vi "main.vi"(11 "client class":refnum<class "client.lvclass">) -> ()   [LabVIEW 2020, in "client.lvclass"]
uses:
  client.lvclass
  shared/message--cluster.ctl
  shared/request--enum.ctl
  client.lvclass/client.ctl
  shared/_JKI_lib_State_Machine.llb/Select State(s)_err__jki_lib_state_machine.vi
panel:
  out "value":T1
  out "error out":errorcluster[](array[cluster])
  in  "Exit":bool
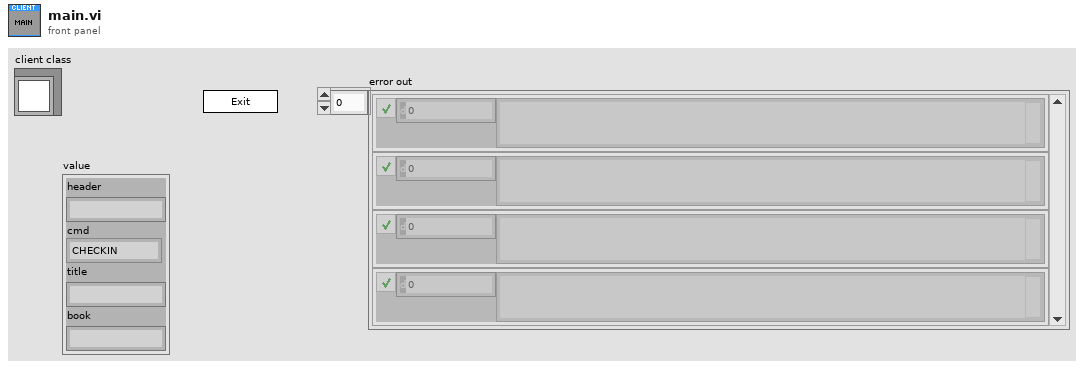
[diagram p1: front panel]
types:
  T1 = typedef "message--cluster.ctl" = cluster{"header":string, "cmd":T2, "title":string, "book":string}
  T2 = typedef "request--enum.ctl" = enum16{"CHECKIN", "CHECKOUT"}
  T3 = enum32{"Invalid", "Standard", "Closed", "Hidden", "Minimized", "Maximized"}
  T4 = enum32{"invalid app kind", "Development System", "Run Time System", "Student Edition", "Embedded LabVIEW", "Evaluation", "Custom"}
  T5 = cluster{"Core":cluster{"Current VI Reference":refnum<vi>, "Close Panel on Exit?":bool}, "client class":refnum<class "client.lvclass">, "TO":i32, "tcp ref":refnum<k5>, "UUID":string, "Book Text":string}
  T6 = cluster{"Current VI Reference":refnum<vi>, "Close Panel on Exit?":bool}
  T7 = cluster{"exit event":refnum<user-event>, "checkout event":refnum<user-event>, "checkin event":refnum<user-event>, "damage event":refnum<user-event>}
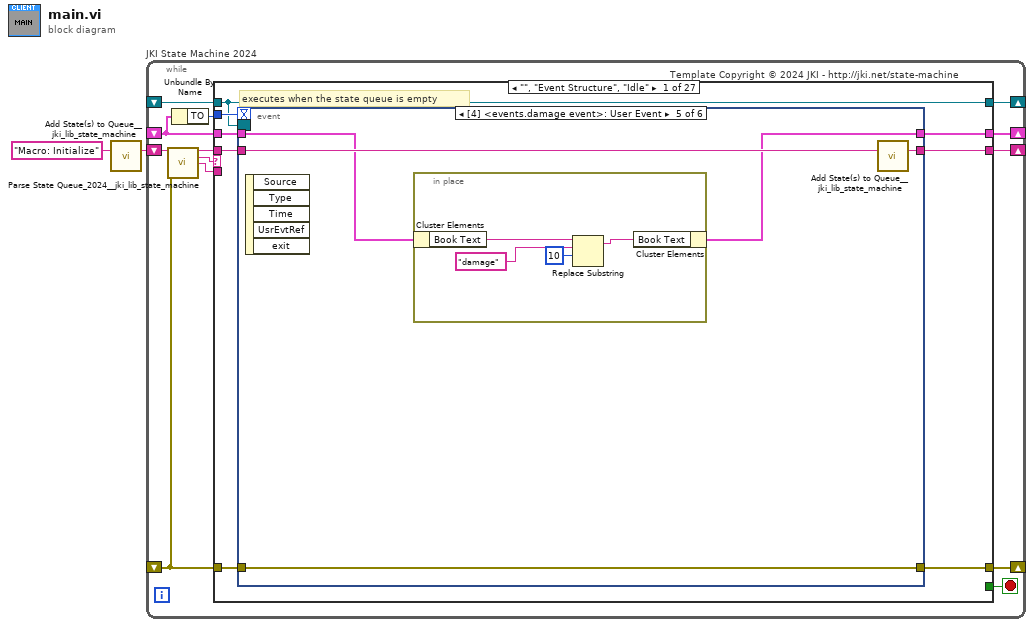
[diagram p0: block diagram]
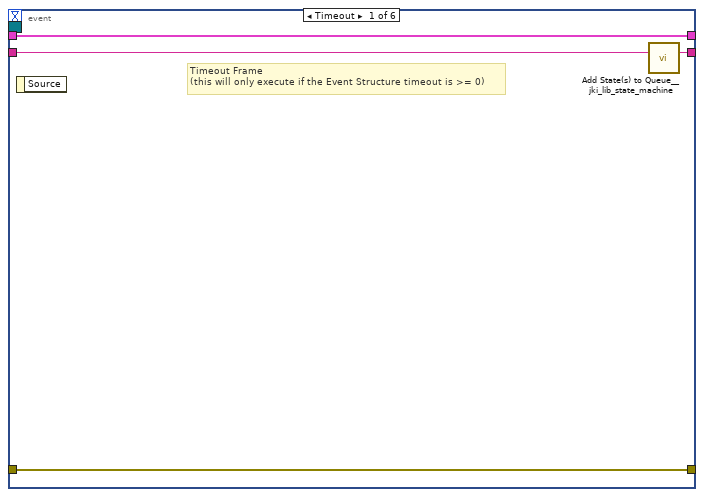
[diagram p2: hidden frame]
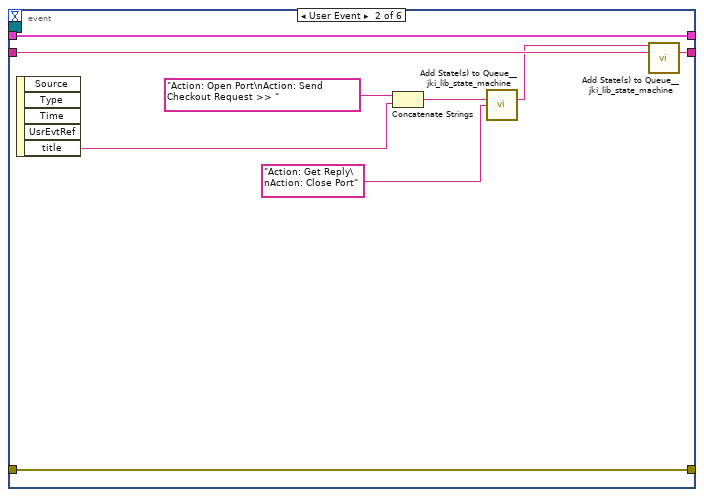
[diagram p3: hidden frame]
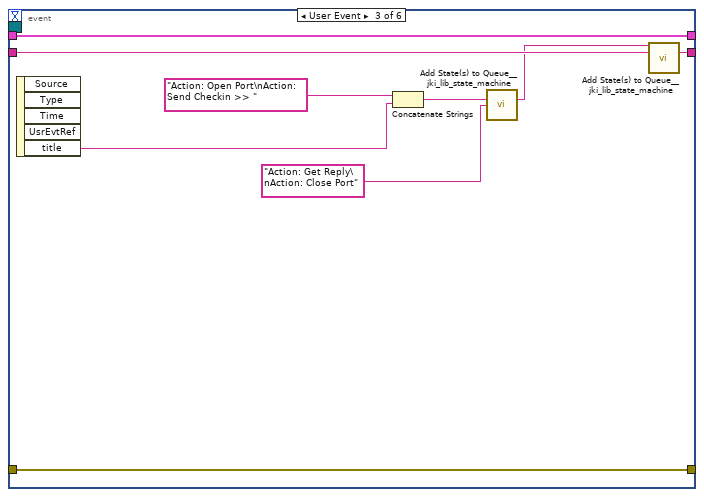
[diagram p4: hidden frame]
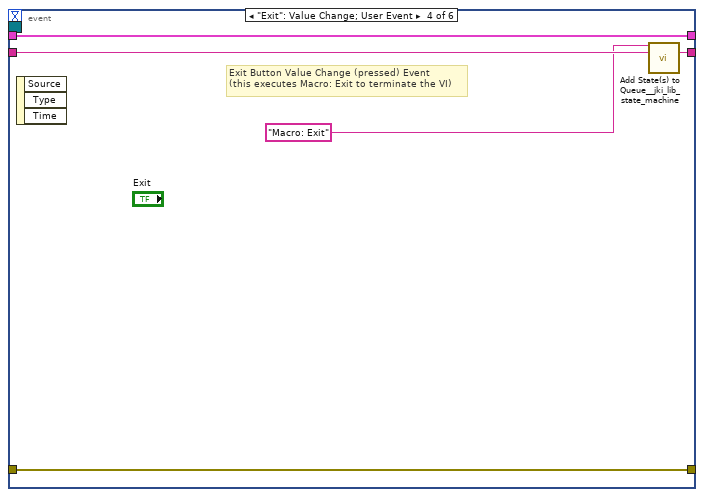
[diagram p5: hidden frame]
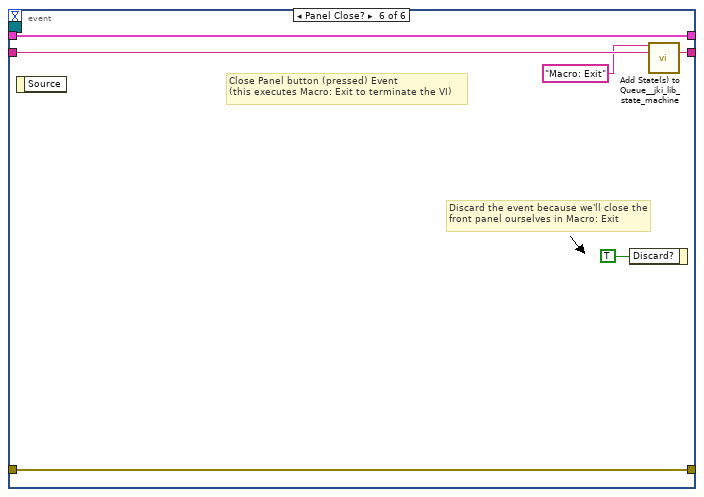
[diagram p6: hidden frame]
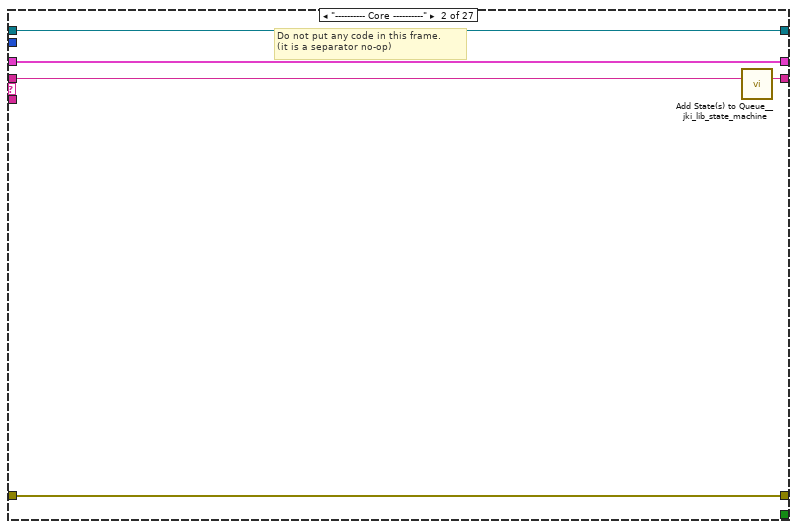
[diagram p7: hidden frame]
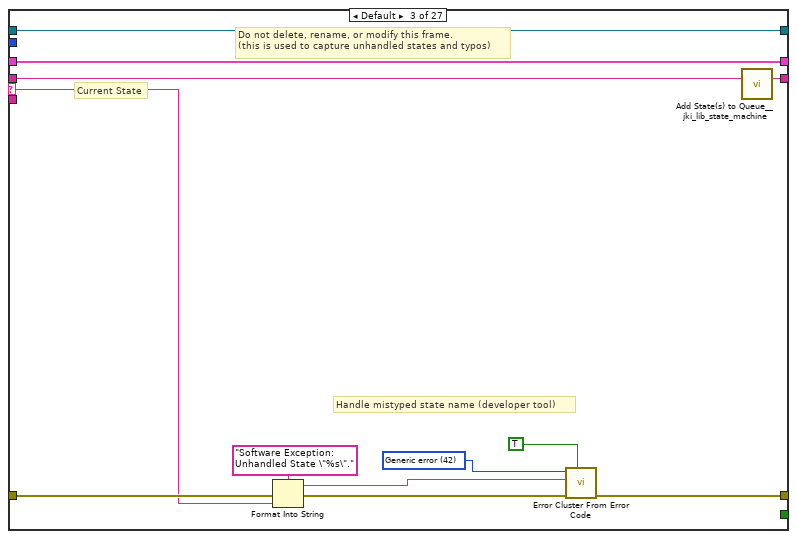
[diagram p8: hidden frame]
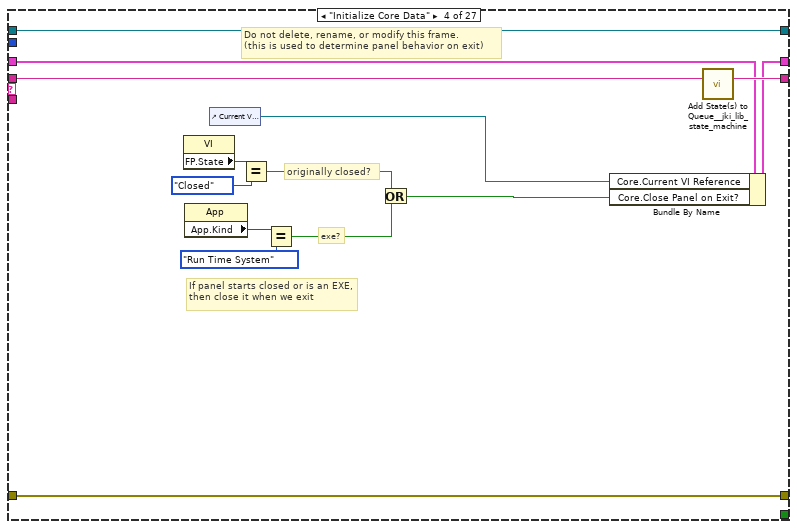
[diagram p9: hidden frame]
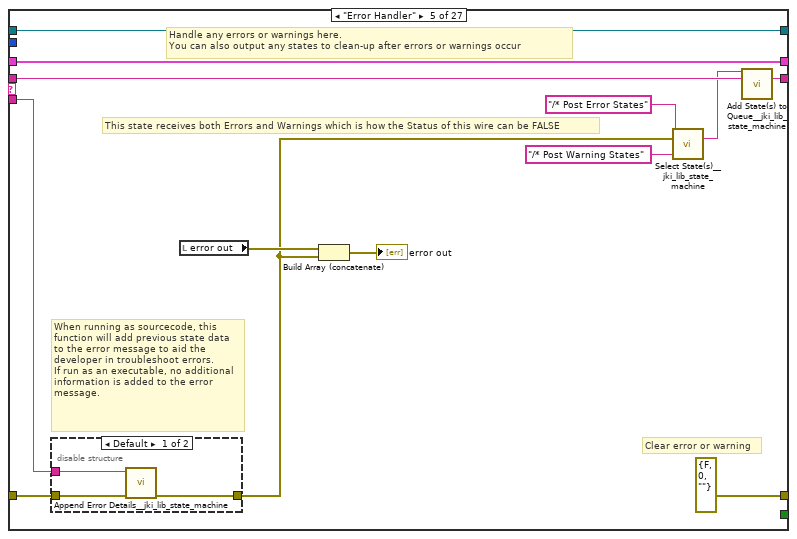
[diagram p10: hidden frame]
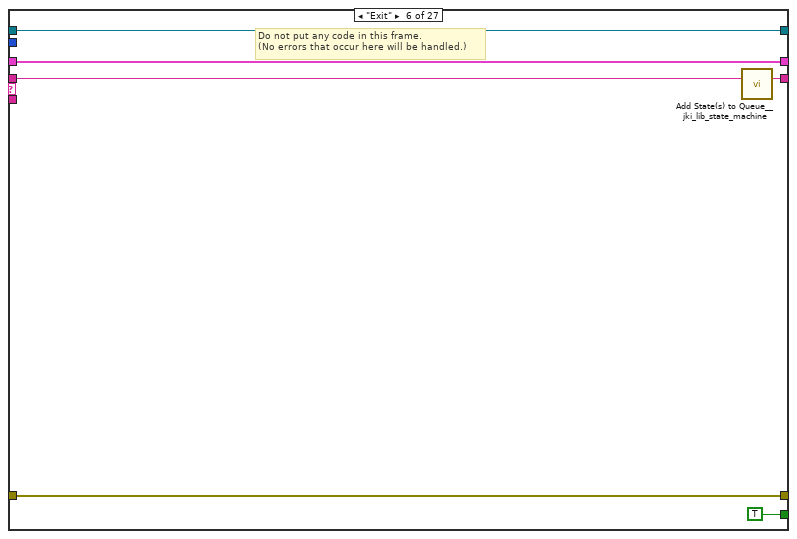
[diagram p12: hidden frame]
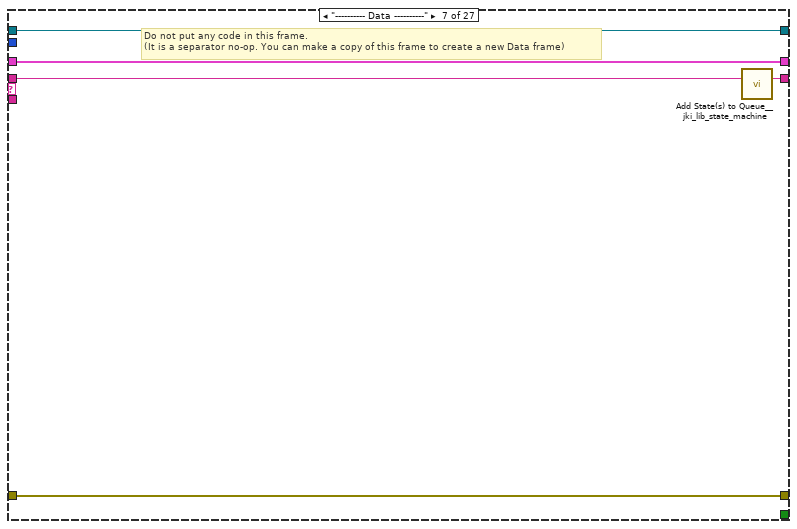
[diagram p13: hidden frame]
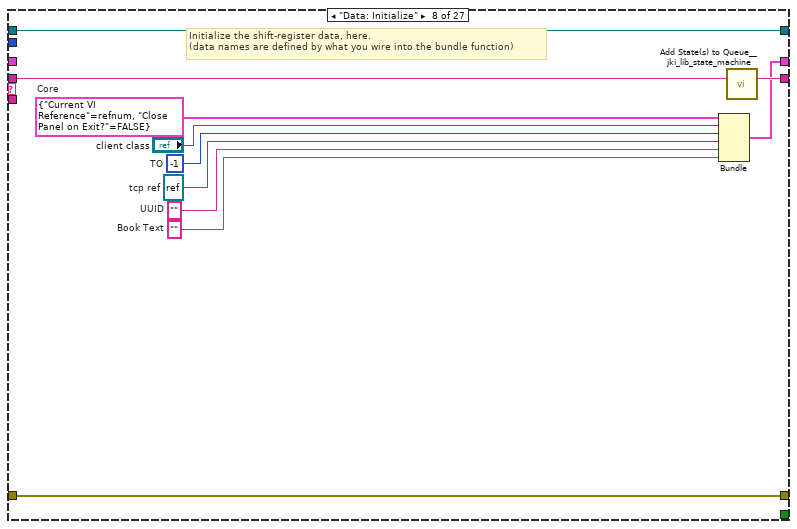
[diagram p14: hidden frame]
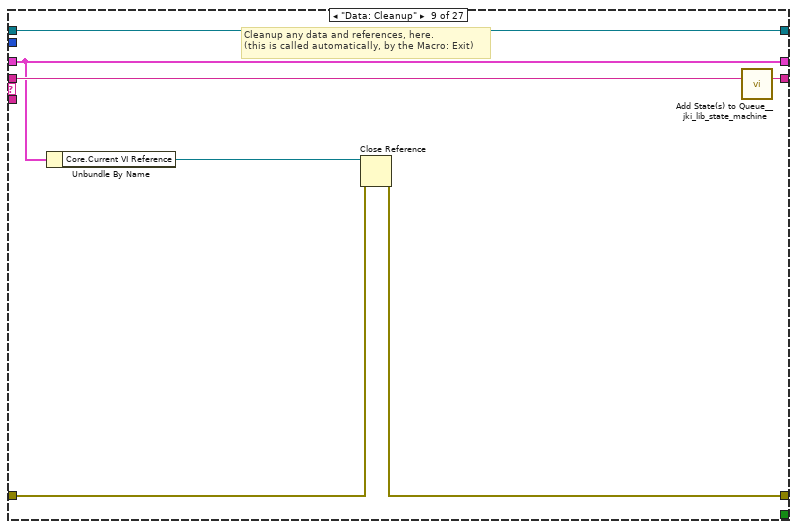
[diagram p15: hidden frame]
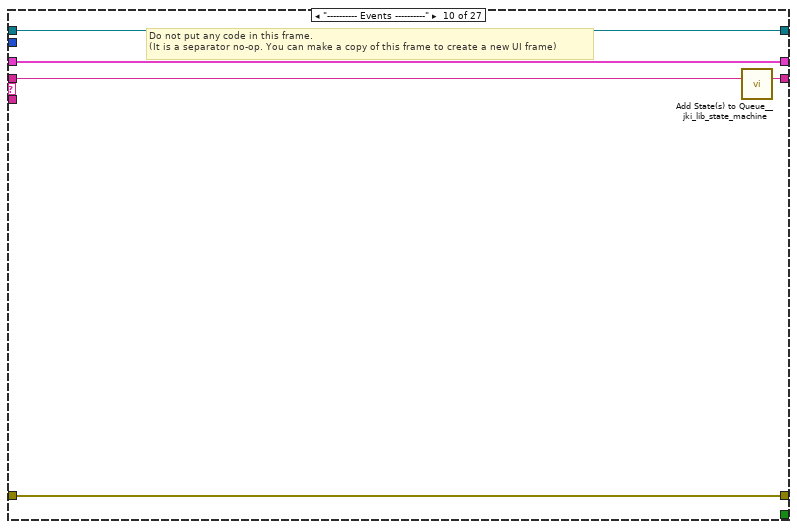
[diagram p16: hidden frame]
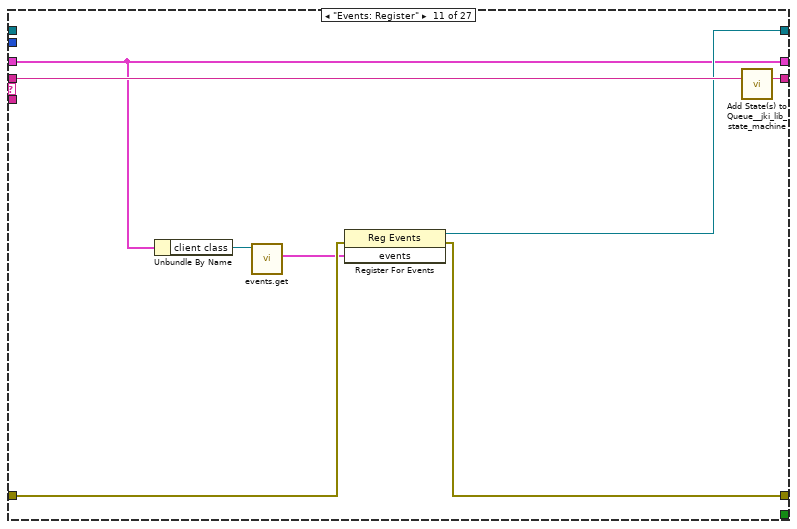
[diagram p17: hidden frame]
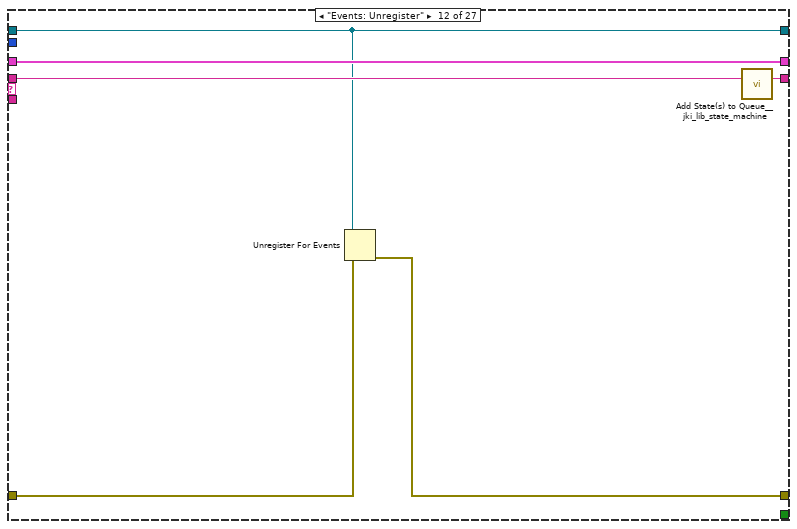
[diagram p18: hidden frame]
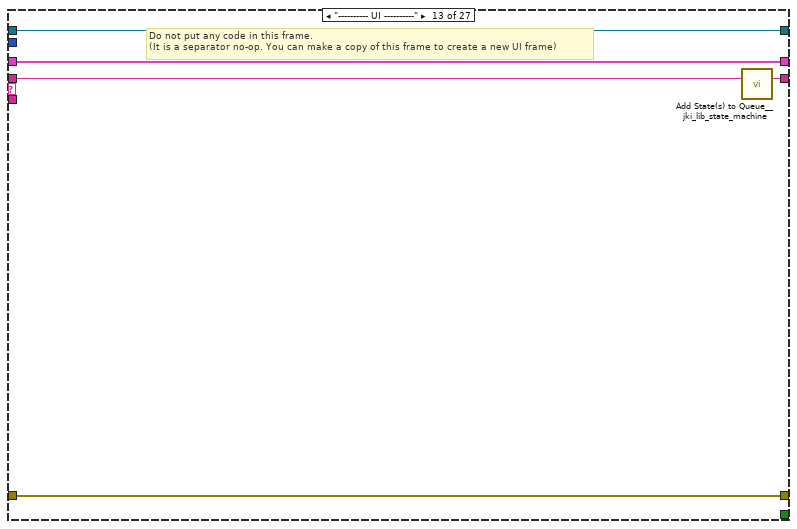
[diagram p19: hidden frame]
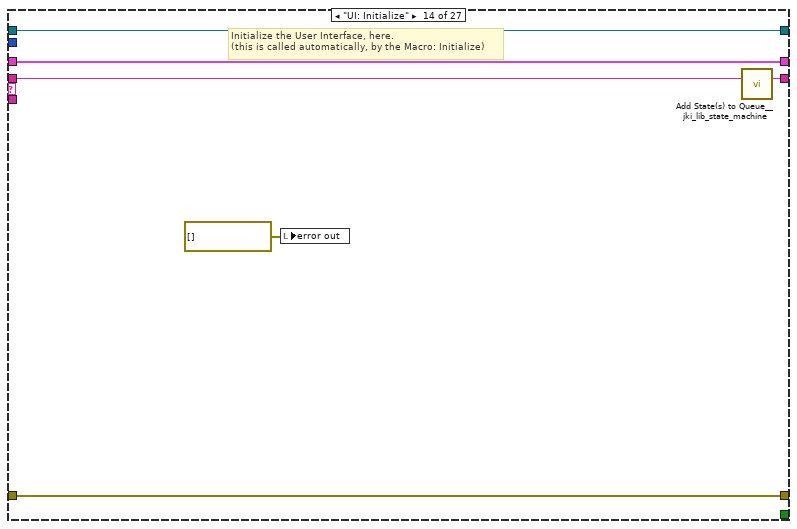
[diagram p20: hidden frame]
diagram:
  n1 = call "Add State(s) to Queue__jki_lib_state_machine.vi"("State(s) in (\"\")"="Macro: Initialize") -> ("States Out"=w2:string)  [unwired: 14 in]
  n2 = while "JKI State Machine 2024" {
    shift-right: [w8] -> _
    shift-left: _ -> [w4]
    shift-right: [w11] -> _
    shift-left: _ -> [w7]
    shift-right: [w10] -> _
    shift-left: w2 -> [w12]
    shift-right: [w6] -> _
    shift-left: _ -> [w5]
    stop <- w9 stop-if-true
    # "Template Copyright © 2024 JKI - http://jki.net/state-machine"
    n3 = call "Parse State Queue_2024__jki_lib_state_machine.vi"("State Queue"=w12, "Error In (no error)"=w7) -> ("Remaining States"=w14:string, "Current State"=w15:string, "Arguments"=w13:string)  [unwired: 11 in]
    n4 = Unbundle By Name(w4) -> ("TO"=w3:i32)
    n5 = case shown="\"\", \"Event Structure\", \"Idle\"" w15 {
      selector: w15 -> [_ _ w72 _ _ _ _ _ _ _ _ _ _ _ _ _ _ _ _ _ _ _ _ _ _ _ _]
      tunnel: w14 -> [w23 w70 w76 w96 w109 w119 w124 w135 w142 w147 w155 w161 w166 w172 w177 w184 w196 w266 w272 w282 w287 w308 w316 w326 w333 w350 w368]
      tunnel: w13 -> [_ _ _ _ w104 _ _ _ _ _ _ _ _ _ _ w179 w190 _ _ _ _ _ _ _ _ w342 w361]
      tunnel: w4 -> [w21 w67 w74 w89 w106 w117 w121 _ w137 w144 w150 w159 w163 w170 w175 w182 w192 w263 w269 w280 w284 w291 w311 w319 w330 w347 w351]
      tunnel: [w20 w68 w78 w93 errorcluster {"status"=FALSE, "code"=0, "source"=""} ("error out") w116 w122 w132 w138 w145 w151 w156 w164 w169 w174 w180 w193 w264 w270 w277 w285 w292 w312 w320 w327 w338 w357] -> w11
      tunnel: w7 -> [w17 w68 w77 w93 w105 w116 w122 w132 w139 w145 w152 w157 w164 w169 w174 w181 w194 w264 w270 w277 w285 w295 w313 w321 w328 w340 w359]
      tunnel: [w22 w69 w75 w95 w108 w118 w123 w134 w141 w146 w154 w160 w165 w171 w176 w183 w195 w265 w271 w281 w286 w307 w315 w325 w332 w349 w367] -> w10
      tunnel: [_ _ _ _ _ TRUE _ _ _ _ _ _ _ _ _ _ _ _ _ _ _ _ _ _ _ _ _] -> w9
      tunnel: [w19 w67 w74 w94 w106 w117 w121 w133 w137 w144 w150 w159 w163 w170 w175 w182 w192 w263 w269 w280 w284 w290 w310 w318 w330 w347 w351] -> w8
      tunnel: w3 -> [w18 _ _ _ _ _ _ _ _ _ _ _ _ _ _ _ _ _ _ _ _ _ _ _ _ _ _]
      tunnel: [w16 w66 w71 w83 w100 w114 w120 w130 w136 w143 w153 w158 w162 w168 w173 w178 w189 w262 w267 w273 w283 w306 w314 w324 w331 w348 w366] -> w6
      tunnel: w5 -> [w16 w66 w71 w83 w100 w114 w120 w130 w136 w143 _ w158 w162 w168 w173 w178 w189 w262 w267 w273 w283 w306 w314 w324 w331 w348 w366]
      frame "", "Event Structure", "Idle" {
        # "executes when the state queue is empty"
        n6 = event shown="[4] <events.damage event>: User Event" {
          selector: w16 -> [_ _ _ _ _ _]
          dyn-events: _ -> [_ _ _ _ _ _]
          timeout: w18 -> [_ _ _ _ _ _]
          tunnel: w23 -> [w27 w36 w45 w50 w55 w65]
          tunnel: [w26 w35 w44 w49 w54 w64] -> w22
          tunnel: w21 -> [w24 w33 w42 w47 w52 w62]
          tunnel: [w25 w34 w43 w48 w53 w63] -> w20
          tunnel: w17 -> [w25 w34 w43 w48 w53 w63]
          tunnel: [w24 w33 w42 w47 w51 w62] -> w19
          event Timeout {
            # "Timeout Frame\n(this will only execute if the Event Structure timeout is >= 0)"
            n7 = event-data() -> ()  [unwired: 1 in, 1 out]
            n8 = call "Add State(s) to Queue__jki_lib_state_machine.vi"("State(s) in (\"\")"=w27) -> ("States Out"=w26:string)  [unwired: 14 in]
          }
          event User Event {
            n9 = event-data() -> ("title"=w31:string)  [unwired: 1 in, 4 out]
            n10 = Concatenate Strings("Action: Open Port\nAction: Send Checkout Request >> ", w31) -> (w30:string)
            n11 = call "Add State(s) to Queue__jki_lib_state_machine.vi"("State(s) in (\"\")"=w30, "State(s) at Back (\"\")"="Action: Get Reply\nAction: Close Port") -> ("States Out"=w28:string)  [unwired: 13 in]
            n12 = call "Add State(s) to Queue__jki_lib_state_machine.vi"("State(s) in Front (\"\")"=w28, "State(s) in (\"\")"=w36) -> ("States Out"=w35:string)  [unwired: 13 in]
          }
          event User Event {
            n13 = event-data() -> ("title"=w40:string)  [unwired: 1 in, 4 out]
            n14 = Concatenate Strings("Action: Open Port\nAction: Send Checkin >> ", w40) -> (w39:string)
            n15 = call "Add State(s) to Queue__jki_lib_state_machine.vi"("State(s) in (\"\")"=w39, "State(s) at Back (\"\")"="Action: Get Reply\nAction: Close Port") -> ("States Out"=w37:string)  [unwired: 13 in]
            n16 = call "Add State(s) to Queue__jki_lib_state_machine.vi"("State(s) in Front (\"\")"=w37, "State(s) in (\"\")"=w45) -> ("States Out"=w44:string)  [unwired: 13 in]
          }
          event "Exit": Value Change; User Event {
            # "Exit Button Value Change (pressed) Event\n(this executes Macro: Exit to terminate the VI)"
            n17 = event-data() -> ()  [unwired: 1 in, 3 out]
            n18 = call "Add State(s) to Queue__jki_lib_state_machine.vi"("State(s) in Front (\"\")"="Macro: Exit", "State(s) in (\"\")"=w50) -> ("States Out"=w49:string)  [unwired: 13 in]
          }
          event User Event {
            n19 = event-data() -> ()  [unwired: 1 in, 5 out]
            n20 = in-place {
              n21 = in-place-cluster #1(w52) -> ("Book Text"=w59:string)
              n22 = Replace Substring(3:10 ("offset (0)"), 4:"damage" ("substring (\"\")"), 5:w59) -> (1:w57:string)  [unwired: 1 in, 1 out]
              n23 = in-place-cluster #1("Book Text"=w57) -> (w51:T5)
            }
            n24 = call "Add State(s) to Queue__jki_lib_state_machine.vi"("State(s) in (\"\")"=w55) -> ("States Out"=w54:string)  [unwired: 14 in]
          }
          event Panel Close? {
            # "Discard the event because we'll close the front panel ourselves in Macro: Exit"
            # "Close Panel button (pressed) Event\n(this executes Macro: Exit to terminate the VI)"
            n25 = event-data() -> ()  [unwired: 1 in, 1 out]
            n26 = event-data("Discard?"=TRUE) -> ()  [unwired: 1 in, 1 out]
            n27 = call "Add State(s) to Queue__jki_lib_state_machine.vi"("State(s) in Front (\"\")"="Macro: Exit", "State(s) in (\"\")"=w65) -> ("States Out"=w64:string)  [unwired: 13 in]
          }
        }
      }
      frame "---------- Core ----------" {
        # "Do not put any code in this frame.\n(it is a separator no-op)"
        n28 = call "Add State(s) to Queue__jki_lib_state_machine.vi"("State(s) in (\"\")"=w70) -> ("States Out"=w69:string)  [unwired: 14 in]
      }
      frame Default {
        w81 = 42 items=["No error", "Argument error", "Memory is full", "Out of zone", "End of file", "File already open", "Generic file I/O error", "File not found", "File permission error", "Disk is full", "Duplicate path", "Too many files open", "System feature not enabled", "Resource file not found", "Cannot add resource", "Resource not found", "Image not found", "Image memory error", "Pen does not exist", "Config type invalid", "Config token not found", "Config parse error", "Config memory error", "Bad external code format", "Bad external code offset", "External code not present", "Null window", "Destroy window error", "Null menu", "Print aborted", "Bad print record", "Print driver error", "Windows error during printing", "Memory error during printing", "Print dialog error", "Generic print error", "Invalid device refnum", "Device not found", "Device parameter error", "Device unit error", "Cannot open device", "Device call aborted", "Generic error", "Cancelled by user", "Object ID too low", "Object ID too high", "Object not in heap", "Unknown heap", "Unknown object (invalid DefProc)", "Unknown object (DefProc not in table)", "Message out of range", "Invalid (null) method", "Unknown message", "Manager call not supported", "Bad address", "Network operation in progress", "Network operation timed out", "Connection is busy", "Network attribute not supported", "Network error", "Address in use", "System out of memory", "Connection aborted", "Connection refused", "Not connected", "Already connected", "Connection closed", "Initialization error (interapplication manager)", "Bad occurrence", "Wait on unbound occurrence handler", "Occurrence queue overflow", "Datalog type conflict", "Unused", "Unrecognized type (interapplication manager)", "Memory corrupt", "Failed to make temporary DLL", "Old CIN version", "Drag socket not found", "Failed to load drop-object", "Failed to register OLE object", "Failed to release OLE object", "Format specifier type mismatch", "Unknown format specifier", "Too few format specifiers", "Too many format specifiers", "Scan failed", "Newer CIN version", "Error converting to variant", "Runtime menu error", "Password tampered", "Variant attribute not found", "Incompatible variant data type", "Event data is not available", "Event Store is not present", "Occurrence is not found", "Event Queue is not created", "Event info is not available", "Refnum passed is NULL", "Error retrieving Class GUID", "Error retrieving CoClass GUID", "Error retrieving TypeLib GUID.", "Bad built application magic bytes.", "Specific driver is different from the specific driver associated with the Logical Name.", "There is no session opened to the class driver.", "Max Error", "MAX - Error with config objects", "MAX - Error loading configuration", "MAX - Group not supported"]
        # "Current State"
        # "Do not delete, rename, or modify this frame.\n(this is used to capture unhandled states and typos)"
        # "Handle mistyped state name (developer tool)"
        n29 = Format Into String(format string="Software Exception: Unhandled State \"%s\"." ("message"), error in=w77, w72) -> (resulting string=w80:string, error out=w79:errorcluster)  [unwired: 1 in]
        n30 = call <vilib>:"Error Cluster From Error Code.vi"("show call chain? (False)"=TRUE, "error in (no error)"=w79, "error message (\"\")"=w80, "error code (0)"=w81) -> ("error out"=w78:errorcluster)  [unwired: 5 in]
        n31 = call "Add State(s) to Queue__jki_lib_state_machine.vi"("State(s) in (\"\")"=w76) -> ("States Out"=w75:string)  [unwired: 14 in]
      }
      frame "Initialize Core Data" {
        # "Do not delete, rename, or modify this frame.\n(this is used to determine panel behavior on exit)"
        # "originally closed?"
        # "exe?"
        # "If panel starts closed or is an EXE, then close it when we exit"
        n32 = property class="VI"() -> ("FP.State"=w86:T3)  [unwired: 2 in, 2 out]
        n33 = property class="App"() -> ("App.Kind"=w92:T4)  [unwired: 2 in, 2 out]
        n34 = control-ref of="Current VI Reference"() -> (w87:refnum<vi>)
        n35 = Equal?(x=w86, y=T3."Closed" ("Front Panel Window:State")) -> (x = y?=w84:bool)
        n36 = Equal?(x=w92, y=T4."Run Time System" ("Application:Kind")) -> (x = y?=w90:bool)
        n37 = Or(x=w84, y=w90) -> (x .or. y?=w88:bool)
        n38 = Bundle By Name(cluster=w89, "Core.Current VI Reference"=w87, "Core.Close Panel on Exit?"=w88) -> (w94:T5)
        n39 = call "Add State(s) to Queue__jki_lib_state_machine.vi"("State(s) in (\"\")"=w96) -> ("States Out"=w95:string)  [unwired: 14 in]
      }
      frame "Error Handler" {
        # "When running as sourcecode, this function will add previous state data to the error message to aid the developer in troubleshoot errors.\nIf run as an executable, no additional information is added to the error message."
        # "This state receives both Errors and Warnings which is how the Status of this wire can be FALSE"
        # "Handle any errors or warnings here.\nYou can also output any states to clean-up after errors or warnings occur"
        # "Clear error or warning"
        n40 = disable-structure shown="Default" {
          disable-tunnel: w105 -> [w112 w113]
          disable-tunnel: w104 -> [w111 _]
          disable-tunnel: [w110 w113] -> w98
          frame condition #0 (active) {
            n41 = call "Append Error Details__jki_lib_state_machine.vi"("error in (no error)"=w112, "Previous State and Argument(s)"=w111) -> ("error out"=w110:errorcluster)  [unwired: 9 in]
          }
          frame condition #1 {
          }
        }
        n42 = local read "error out"() -> (w99:errorcluster[])
        n43 = Build Array (concatenate)(w99, w98) -> (→"error out":errorcluster[])
        n44 = call-poly "Select State(s)__jki_lib_state_machine.vi"("State(s) if True (\"\")"="/* Post Error States", "Select"=w98, "State(s) if False (\"\")"="/* Post Warning States") -> ("States Out"=w102:string)  [unwired: 12 in]
        n45 = call "Add State(s) to Queue__jki_lib_state_machine.vi"("State(s) in Front (\"\")"=w102, "State(s) in (\"\")"=w109) -> ("States Out"=w108:string)  [unwired: 13 in]
      }
      frame "Exit" {
        # "Do not put any code in this frame.\n(No errors that occur here will be handled.)"
        n46 = call "Add State(s) to Queue__jki_lib_state_machine.vi"("State(s) in (\"\")"=w119) -> ("States Out"=w118:string)  [unwired: 14 in]
      }
      frame "---------- Data ----------" {
        # "Do not put any code in this frame.\n(It is a separator no-op. You can make a copy of this frame to create a new Data frame)"
        n47 = call "Add State(s) to Queue__jki_lib_state_machine.vi"("State(s) in (\"\")"=w124) -> ("States Out"=w123:string)  [unwired: 14 in]
      }
      frame "Data: Initialize" {
        w125 = ""  # Book Text
        w126 = ""  # UUID
        w127 = refnum<k5> refnum  # tcp ref
        w128 = -1  # TO
        w131 = T6 {"Current VI Reference"=refnum, "Close Panel on Exit?"=FALSE}  # Core
        # "Initialize the shift-register data, here.\n(data names are defined by what you wire into the bundle function)"
        n48 = Bundle("Core"=w131, "client class"="client class", "TO"=w128, "tcp ref"=w127, "UUID"=w126, "Book Text"=w125) -> (w133:T5)  [unwired: 1 in]
        n49 = call "Add State(s) to Queue__jki_lib_state_machine.vi"("State(s) in (\"\")"=w135) -> ("States Out"=w134:string)  [unwired: 14 in]
      }
      frame "Data: Cleanup" {
        # "Cleanup any data and references, here.\n(this is called automatically, by the Macro: Exit)"
        n50 = Unbundle By Name(w137) -> ("Core.Current VI Reference"=w140:refnum<vi>)
        n51 = Close Reference(reference=w140, error in (no error)=w139) -> (error out=w138:errorcluster)
        n52 = call "Add State(s) to Queue__jki_lib_state_machine.vi"("State(s) in (\"\")"=w142) -> ("States Out"=w141:string)  [unwired: 14 in]
      }
      frame "---------- Events ----------" {
        # "Do not put any code in this frame.\n(It is a separator no-op. You can make a copy of this frame to create a new UI frame)"
        n53 = call "Add State(s) to Queue__jki_lib_state_machine.vi"("State(s) in (\"\")"=w147) -> ("States Out"=w146:string)  [unwired: 14 in]
      }
      frame "Events: Register" {
        n54 = Unbundle By Name(w150) -> ("client class"=w149:refnum<class "client.lvclass">)
        n55 = call "events.get.vi"("client in"=w149) -> ("events"=w148:T7)  [unwired: 9 in, 1 out]
        n56 = register-events(error in=w152, w148) -> (reference out=w153:refnum<event-registration>, error out=w151:errorcluster)  [unwired: 1 in]
        n57 = call "Add State(s) to Queue__jki_lib_state_machine.vi"("State(s) in (\"\")"=w155) -> ("States Out"=w154:string)  [unwired: 14 in]
      }
      frame "Events: Unregister" {
        n58 = Unregister For Events(event registration refnum=w158, error in=w157) -> (error out=w156:errorcluster)
        n59 = call "Add State(s) to Queue__jki_lib_state_machine.vi"("State(s) in (\"\")"=w161) -> ("States Out"=w160:string)  [unwired: 14 in]
      }
      frame "---------- UI ----------" {
        # "Do not put any code in this frame.\n(It is a separator no-op. You can make a copy of this frame to create a new UI frame)"
        n60 = call "Add State(s) to Queue__jki_lib_state_machine.vi"("State(s) in (\"\")"=w166) -> ("States Out"=w165:string)  [unwired: 14 in]
      }
      frame "UI: Initialize" {
        # "Initialize the User Interface, here.\n(this is called automatically, by the Macro: Initialize)"
        n61 = local write "error out"(errorcluster[] [] ("error out")) -> ()
        n62 = call "Add State(s) to Queue__jki_lib_state_machine.vi"("State(s) in (\"\")"=w172) -> ("States Out"=w171:string)  [unwired: 14 in]
      }
      frame "UI: Uninitialize" {
        # "Cleanup the User Interface, here.\n(this is called automatically, by the Macro: Exit)"
        n63 = call "Add State(s) to Queue__jki_lib_state_machine.vi"("State(s) in (\"\")"=w177) -> ("States Out"=w176:string)  [unwired: 14 in]
      }
      frame "UI: Cursor Set" {
        # "Argument"
        # "Set and Unset Cursor Busy.\n(Usage: \"UI: Cursor Set >> Busy|Idle\")"
        n64 = case shown="\"Idle\", Default" w179 {
          tunnel: w181 -> [w186 w188]
          tunnel: [w185 w187] -> w180
          frame "Idle", Default {
            n65 = call <vilib>:"Unset Busy.vi"("error in (no error)"=w186) -> ("error out"=w185:errorcluster)  [unwired: 10 in]
          }
          frame "Busy" {
            n66 = call <vilib>:"Set Busy.vi"("error in (no error)"=w188) -> ("error out"=w187:errorcluster)  [unwired: 9 in, 1 out]
          }
        }
        n67 = call "Add State(s) to Queue__jki_lib_state_machine.vi"("State(s) in (\"\")"=w184) -> ("States Out"=w183:string)  [unwired: 14 in]
      }
      frame "UI: Front Panel State" {
        # "Argument"
        # "Set Front Panel Open or Closed\n(Usage: \"UI: Front Panel State >> Open|Close\")"
        n68 = Unbundle By Name(w192) -> ("Core.Current VI Reference"=w191:refnum<vi>)
        n69 = case shown="\"Minimize\", \"Minimized\"" w190 {
          tunnel: w194 -> [w202 w217 w228 w241 w254]
          tunnel: [w204 w218 w230 w243 w256] -> w193
          tunnel: w191 -> [w203 w215 w229 w242 w255]
          frame "Open", "Standard", Default {
            w197 = T3."Standard" ("State")
            n70 = property class="VI"(reference=w203, error in=w202) -> (reference out=w200:refnum<vi>, error out=w201:errorcluster, "FP.State"=w199:T3)
            n71 = Not Equal?(x=w199, y=w197) -> (x != y?=w198:bool)
            n72 = case shown="True" w198 {
              tunnel: [w208 w210] -> w204
              tunnel: w201 -> [w207 w210]
              tunnel: w200 -> [w206 _]
              tunnel: w197 -> [w205 _]
              frame True {
                n73 = invoke class="VI" method="FP.Open"(reference=w206, error in=w207, "Activate"=TRUE, "State"=w205) -> (error out=w208:errorcluster)  [unwired: 1 in, 4 out]
              }
              frame False {
              }
            }
          }
          frame "Close", "Closed" {
            n74 = property class="VI"(reference=w215, error in=w217) -> (reference out=w214:refnum<vi>, error out=w216:errorcluster, "FP.State"=w212:T3)
            n75 = Not Equal?(x=w212, y=T3."Closed" ("Front Panel Window:State")) -> (x != y?=w211:bool)
            n76 = case shown="True" w211 {
              tunnel: [w219 w222] -> w218
              tunnel: w216 -> [w219 w221]
              tunnel: w214 -> [_ w220]
              frame False {
              }
              frame True {
                n77 = invoke class="VI" method="FP.Close"(reference=w220, error in=w221) -> (error out=w222:errorcluster)  [unwired: 1 in, 2 out]
              }
            }
          }
          frame "Hidden", "Hide" {
            w223 = T3."Hidden" ("State")
            n78 = property class="VI"(reference=w229, error in=w228) -> (reference out=w226:refnum<vi>, error out=w227:errorcluster, "FP.State"=w225:T3)
            n79 = Not Equal?(x=w225, y=w223) -> (x != y?=w224:bool)
            n80 = case shown="True" w224 {
              tunnel: [w234 w235] -> w230
              tunnel: w227 -> [w233 w235]
              tunnel: w226 -> [w232 _]
              tunnel: w223 -> [w231 _]
              frame True {
                n81 = invoke class="VI" method="FP.Open"(reference=w232, error in=w233, "State"=w231) -> (error out=w234:errorcluster)  [unwired: 2 in, 4 out]
              }
              frame False {
              }
            }
          }
          frame "Minimize", "Minimized" {
            w236 = T3."Minimized" ("State")
            n82 = property class="VI"(reference=w242, error in=w241) -> (reference out=w239:refnum<vi>, error out=w240:errorcluster, "FP.State"=w238:T3)
            n83 = Not Equal?(x=w238, y=w236) -> (x != y?=w237:bool)
            n84 = case shown="True" w237 {
              tunnel: [w247 w248] -> w243
              tunnel: w240 -> [w246 w248]
              tunnel: w239 -> [w245 _]
              tunnel: w236 -> [w244 _]
              frame True {
                n85 = invoke class="VI" method="FP.Open"(reference=w245, error in=w246, "State"=w244) -> (error out=w247:errorcluster)  [unwired: 2 in, 4 out]
              }
              frame False {
              }
            }
          }
          frame "Maximize", "Maximized" {
            w249 = T3."Maximized" ("State")
            n86 = property class="VI"(reference=w255, error in=w254) -> (reference out=w252:refnum<vi>, error out=w253:errorcluster, "FP.State"=w251:T3)
            n87 = Not Equal?(x=w251, y=w249) -> (x != y?=w250:bool)
            n88 = case shown="True" w250 {
              tunnel: [w260 w261] -> w256
              tunnel: w253 -> [w259 w261]
              tunnel: w252 -> [w258 _]
              tunnel: w249 -> [w257 _]
              frame True {
                n89 = invoke class="VI" method="FP.Open"(reference=w258, error in=w259, "State"=w257) -> (error out=w260:errorcluster)  [unwired: 2 in, 4 out]
              }
              frame False {
              }
            }
          }
        }
        n90 = call "Add State(s) to Queue__jki_lib_state_machine.vi"("State(s) in (\"\")"=w196) -> ("States Out"=w195:string)  [unwired: 14 in]
      }
      frame "---------- Macro ----------" {
        # "Do not put any code in this frame.\n(It is a separator no-op. You can make a copy of this frame to create a new Macro frame)"
        n91 = call "Add State(s) to Queue__jki_lib_state_machine.vi"("State(s) in (\"\")"=w266) -> ("States Out"=w265:string)  [unwired: 14 in]
      }
      frame "Macro: Initialize" {
        # "Initialization Macro\n(This is called once, when the VI starts)"
        n92 = call "Add State(s) to Queue__jki_lib_state_machine.vi"("State(s) in Front (\"\")"="Data: Initialize\nInitialize Core Data\nEvents: Register\nUI: Initialize\nUI: Front Panel State >> Open\nAction: Create UUID", "State(s) in (\"\")"=w272) -> ("States Out"=w271:string)  [unwired: 13 in]
      }
      frame "Macro: Exit" {
        # "Exit Macro\n(This is called once, when the VI exits)"
        n93 = Unbundle By Name(w280) -> ("Core.Close Panel on Exit?"=w275:bool)
        n94 = call "Conditional State String__jki_lib_state_machine.vi"("Do State(s)?"=w275, "State"="UI: Front Panel State >> Close") -> ("State Out"=w274:string)  [unwired: 7 in]
        n95 = call "Add State(s) to Queue__jki_lib_state_machine.vi"("State(s) in (\"\")"=w274, "State(s) at Back (\"\")"="UI: Uninitialize\nData: Cleanup\nEvents: Unregister\nExit") -> ("States Out"=w278:string)  [unwired: 13 in]
        n96 = call "Add State(s) to Queue__jki_lib_state_machine.vi"("State(s) in Front (\"\")"=w278, "State(s) in (\"\")"=w282) -> ("States Out"=w281:string)  [unwired: 13 in]
      }
      frame "---------- Action  ----------" {
        # "Template Separator\n(You can make a copy of, or modify, this frame)"
        n97 = call "Add State(s) to Queue__jki_lib_state_machine.vi"("State(s) in (\"\")"=w287) -> ("States Out"=w286:string)  [unwired: 14 in]
      }
      frame "Action: Get Reply" {
        w300 = 1000  # timout
        w301 = 4  # I32
        n98 = Unbundle By Name(w291) -> ("tcp ref"=w299:refnum<k5>, "client class"=w294:refnum<class "client.lvclass">)
        n99 = TCP Read(connection ID=w299, bytes to read=w301, error in (no error)=w295, 9:w300) -> (connection ID out=w302:refnum<k5>, data out=w305:string, error out=w304:errorcluster)  [unwired: 1 out]
        n100 = Type Cast(type=w301, x=w305) -> (*(type *) &x=w303:i32)
        n101 = TCP Read(connection ID=w302, bytes to read=w303, error in (no error)=w304, 9:w300) -> (data out=w298:string, error out=w296:errorcluster)  [unwired: 2 out]
        n102 = Unflatten From String(type=T1 {"header"="", "cmd"=enum."CHECKIN", "title"="", "book"=""} ("request"), binary string=w298, error in (no error)=w296) -> (value=w288:T1, error out=w293:errorcluster)  [unwired: 2 in, 1 out]
        "value" <- w288
        n103 = Unbundle By Name(w288) -> ("book"=w289:string)
        n104 = Bundle By Name(cluster=w291, "Book Text"=w289) -> (w290:T5)
        n105 = call "send_reply.vi"("error in (no error)"=w293, "message"=w288, "client in"=w294) -> ("error out"=w292:errorcluster)  [unwired: 7 in, 1 out]
        n106 = call "Add State(s) to Queue__jki_lib_state_machine.vi"("State(s) in (\"\")"=w308) -> ("States Out"=w307:string)  [unwired: 14 in]
      }
      frame "Action: Create UUID" {
        n107 = call "generate.UUID.vi"("error in (no error)"=w313) -> ("error out"=w312:errorcluster, "UUID"=w309:string)  [unwired: 9 in]
        n108 = Bundle By Name(cluster=w311, "UUID"=w309) -> (w310:T5)
        n109 = call "Add State(s) to Queue__jki_lib_state_machine.vi"("State(s) in (\"\")"=w316) -> ("States Out"=w315:string)  [unwired: 14 in]
      }
      frame "Action: Open Port" {
        w322 = 30000  # timeout ms
        w323 = u16 6340  # port
        n110 = TCP Open Connection(remote port or service name=w323, timeout ms (60000)=w322, error in (no error)=w321) -> (connection ID=w317:refnum<k5>, error out=w320:errorcluster)  [unwired: 2 in]
        n111 = Bundle By Name(cluster=w319, "tcp ref"=w317) -> (w318:T5)
        n112 = call "Add State(s) to Queue__jki_lib_state_machine.vi"("State(s) in (\"\")"=w326) -> ("States Out"=w325:string)  [unwired: 14 in]
      }
      frame "Action: Close Port" {
        n113 = Unbundle By Name(w330) -> ("tcp ref"=w329:refnum<k5>)
        n114 = TCP Close Connection(connection ID=w329, error in (no error)=w328) -> (error out=w327:errorcluster)  [unwired: 1 in, 1 out]
        n115 = call "Add State(s) to Queue__jki_lib_state_machine.vi"("State(s) in (\"\")"=w333) -> ("States Out"=w332:string)  [unwired: 14 in]
      }
      frame "Action: Send Checkout Request" {
        n116 = Unbundle By Name(w347) -> ("tcp ref"=w346:refnum<k5>, "UUID"=w344:string)
        n117 = Bundle By Name(cluster=T1 {"header"="", "cmd"=enum."CHECKIN", "title"="", "book"=""} ("request"), "header"=w344, "cmd"=request--enum."CHECKOUT", "title"=w342) -> (w341:T1)
        n118 = Flatten To String(anything=w341, error in (no error)=w340) -> (data string=w335:string, error out=w339:errorcluster)  [unwired: 2 in, 1 out]
        n119 = String Length(string=w335) -> (length=w337:i32)
        n120 = Type Cast(x=w337) -> (*(type *) &x=w336:string)  [unwired: 1 in]
        n121 = Concatenate Strings(w336, w335) -> (w334:string)
        n122 = TCP Write(connection ID=w346, data in=w334, error in (no error)=w339) -> (error out=w338:errorcluster)  [unwired: 1 in, 2 out]
        n123 = call "Add State(s) to Queue__jki_lib_state_machine.vi"("State(s) in (\"\")"=w350) -> ("States Out"=w349:string)  [unwired: 14 in]
      }
      frame "Action: Send Checkin" {
        n124 = Unbundle By Name(w351) -> ("tcp ref"=w365:refnum<k5>, "UUID"=w363:string, "Book Text"=w352:string)
        n125 = Bundle By Name(cluster=T1 {"header"="", "cmd"=enum."CHECKIN", "title"="", "book"=""} ("request"), "header"=w363, "cmd"=request--enum."CHECKIN", "title"=w361, "book"=w352) -> (w360:T1)
        n126 = Flatten To String(anything=w360, error in (no error)=w359) -> (data string=w354:string, error out=w358:errorcluster)  [unwired: 2 in, 1 out]
        n127 = String Length(string=w354) -> (length=w356:i32)
        n128 = Type Cast(x=w356) -> (*(type *) &x=w355:string)  [unwired: 1 in]
        n129 = Concatenate Strings(w355, w354) -> (w353:string)
        n130 = TCP Write(connection ID=w365, data in=w353, error in (no error)=w358) -> (error out=w357:errorcluster)  [unwired: 1 in, 2 out]
        n131 = call "Add State(s) to Queue__jki_lib_state_machine.vi"("State(s) in (\"\")"=w368) -> ("States Out"=w367:string)  [unwired: 14 in]
      }
    }
  }
